vi "FPGAPressure.vi"() -> ()   [LabVIEW 2019]
uses:
  <vilib>/rvi/eio/common/nirviEmuTemplateMethod_errors.vi
  <vilib>/eio/EIONode/EIONode.xnode
panel:
  out "Pressure Out (bar)":sgl
  out "Pressure In (bar)":sgl
  out "Mod3-9203/AI2":sgl
  out "Mod3-9203/AI1":sgl
  # "READ Pressure Sensors"
  # "Honeywell MLH08KPSB01B"
  # "(Amps)"
  # "(Amps)"
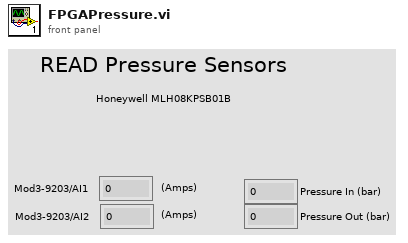
[diagram p1: front panel]
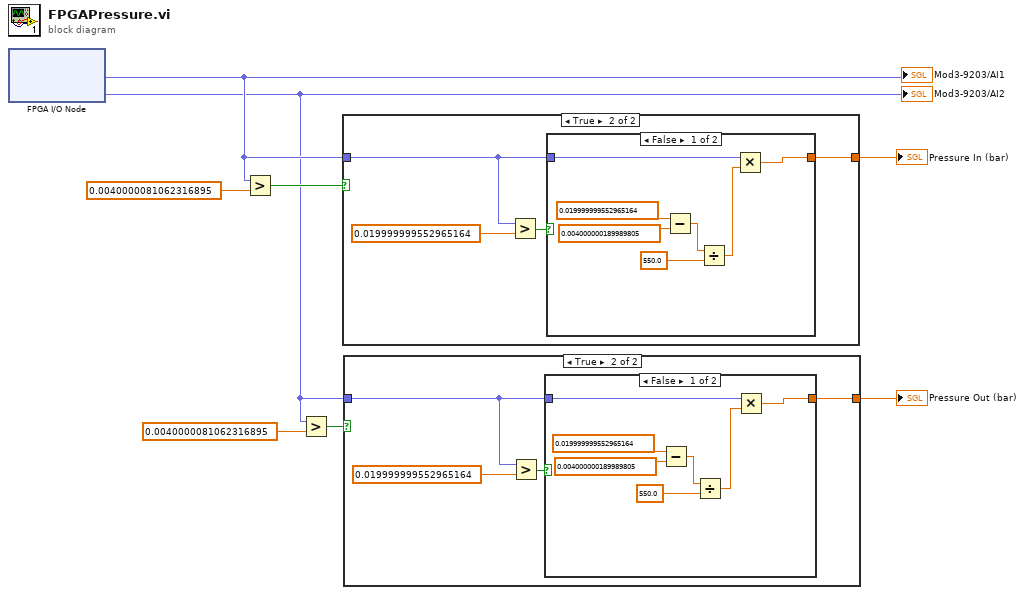
[diagram p0: block diagram]
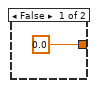
[diagram p2: hidden frame]
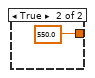
[diagram p3: hidden frame]
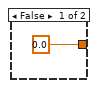
[diagram p4: hidden frame]
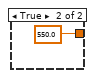
[diagram p5: hidden frame]
diagram:
  n1 = xnode "FPGA I/O Node"() -> ("Mod3/AI1"=w6:fxp<+/-,21,-4>, "Mod3/AI2"=w1:fxp<+/-,21,-4>)  [unwired: 2 in, 2 out]
  "Mod3-9203/AI1" <- w6
  "Mod3-9203/AI2" <- w1
  n2 = Greater?(x=w6, y=sgl 0.004000008) -> (0:w7:bool)
  n3 = Greater?(x=w1, y=sgl 0.004000008) -> (0:w3:bool)
  n4 = case shown="True" w7 {
    tunnel: w6 -> [_ w10]
    tunnel: [sgl 0.0 w11] -> w5
    frame False {
    }
    frame True {
      n5 = Greater?(x=w10, y=sgl 0.02) -> (0:w13:bool)
      n6 = case shown="False" w13 {
        tunnel: [w19 sgl 550.0] -> w11
        tunnel: w10 -> [w20 _]
        frame False {
          n7 = Subtract(x=sgl 0.02, y=sgl 0.004) -> (x-y=w18:sgl)
          n8 = Divide(x=w18, y=sgl 550.0 ("x")) -> (x/y=w14:sgl)
          n9 = Multiply(x=w20, y=w14) -> (x*y=w19:sgl)
        }
        frame True {
        }
      }
    }
  }
  "Pressure In (bar)" <- w5
  n10 = case shown="True" w3 {
    tunnel: w1 -> [_ w23]
    tunnel: [sgl 0.0 w24] -> w2
    frame False {
    }
    frame True {
      n11 = Greater?(x=w23, y=sgl 0.02) -> (0:w26:bool)
      n12 = case shown="False" w26 {
        tunnel: [w29 sgl 550.0] -> w24
        tunnel: w23 -> [w30 _]
        frame False {
          n13 = Subtract(x=sgl 0.02, y=sgl 0.004) -> (x-y=w33:sgl)
          n14 = Divide(x=w33, y=sgl 550.0 ("x")) -> (x/y=w28:sgl)
          n15 = Multiply(x=w30, y=w28) -> (x*y=w29:sgl)
        }
        frame True {
        }
      }
    }
  }
  "Pressure Out (bar)" <- w2
